vi "Write Register (U8).vi"(0 "SLSC Interface in":refnum<class "SLSC Interface.lvclass">, 5 "device":refnum<k21>="$DefaultDevices", 7 "register address":u32 format="%.0x", 9 "data in":u8 format="%.0x", 11 "error in (no error)":errorcluster) -> (4 "SLSC Interface out":refnum<class "SLSC Interface.lvclass">, 6 "device out":refnum<k21>, 8 "next register address":u32 format="%.0x", 15 "error out":errorcluster)   [LabVIEW 2015, in "SLSC Interfaces.lvlib" / "SLSC Interface.lvclass"]
uses:
  SLSC Interface.lvclass
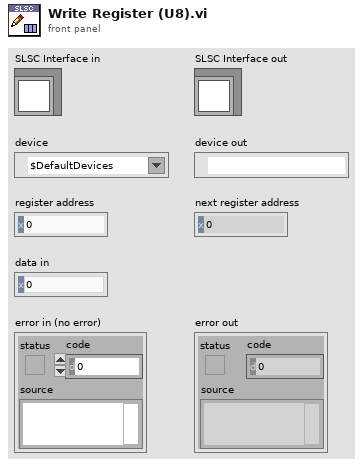
[diagram p1: front panel]
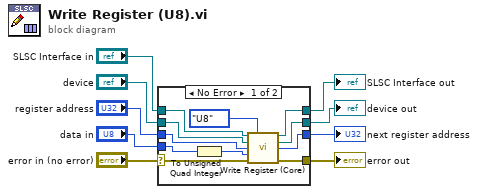
[diagram p0: block diagram]
diagram:
  n1 = case shown="No Error" "error in (no error)" {
    selector: "error in (no error)" -> [w18 w24]
    tunnel: [w17 w24] -> w8
    tunnel: [w19 w23] -> w6
    tunnel: "SLSC Interface in" -> [w20 w23]
    tunnel: "register address" -> [w12 w22]
    tunnel: [w15 w21] -> w4
    tunnel: [w14 w22] -> w3
    tunnel: "device" -> [w13 w21]
    tunnel: "data in" -> [w11 _]
    frame No Error {
      n2 = To Unsigned Quad Integer(1:w11) -> (0:w10:u64)
      n3 = call-dynamic "Write Register (Core).vi"("SLSC Interface in"=w20, "type"=enum16{"U8", "U16", "U32", "U64"}."U8" ("size"), "device"=w13, "register address"=w12, "data"=w10, "error in (no error)"=w18) -> ("SLSC Interface out"=w19:refnum<class "SLSC Interface.lvclass">, "device out"=w15:refnum<k21>, "next register address"=w14:u32, "error out"=w17:errorcluster)  [unwired: 6 in]
    }
    frame Error {
    }
  }
  "error out" <- w8
  "SLSC Interface out" <- w6
  "device out" <- w4
  "next register address" <- w3
